vi "Puzzle 3-2.vi"() -> ()   [LabVIEW 2022 SP3]
panel:
  out "Array 4":cluster{i32, i32}[](array[cluster])
  out "sum":i32
  out "Array 3":cluster{i32, i32}[](array[cluster])
  out "Array 2":enum16{"Letter", "Number", "Symbol", "Dot"}[][](array[ring])
  out "Array":string[][](array[string])
  in  "delimited string":string
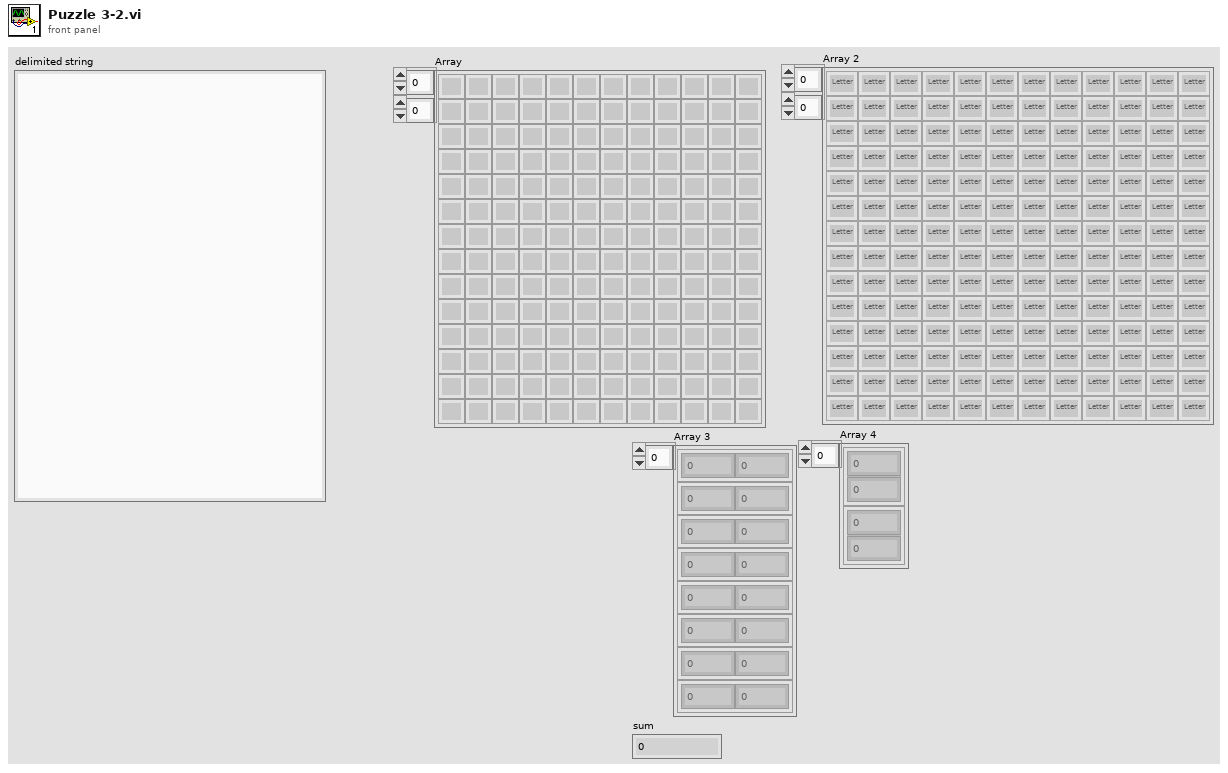
[diagram p1: front panel]
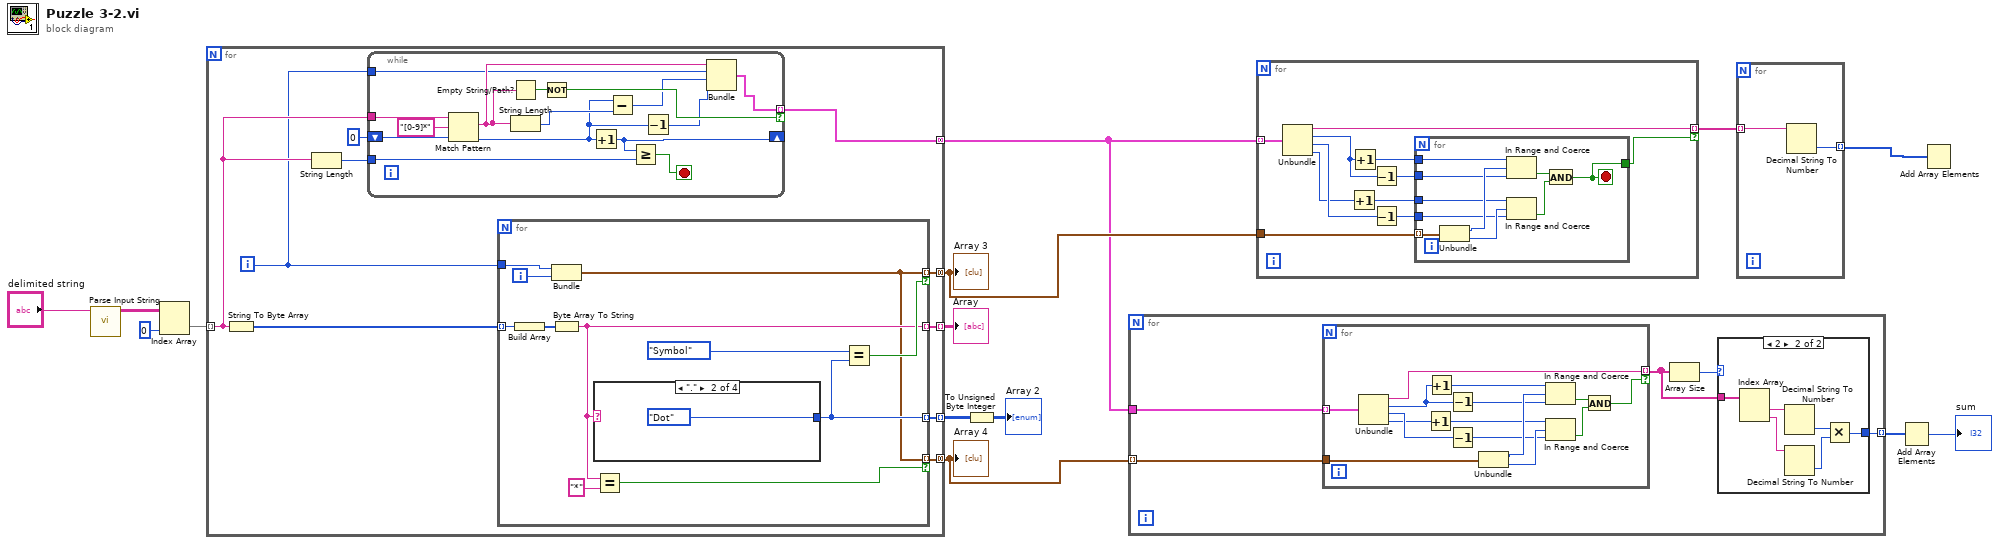
[diagram p0: block diagram]
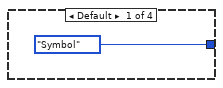
[diagram p3: hidden frame]
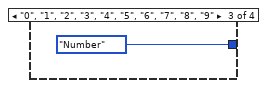
[diagram p4: hidden frame]
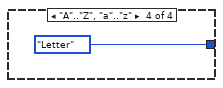
[diagram p5: hidden frame]
diagram:
  n1 = call "Parse Input String.vi"("delimited string"="delimited string") -> ("parsed string"=w13:string[][])  [unwired: 10 in]
  n2 = Index Array(array=w13, index (col)=0 ("disabled index (col)")) -> (element=w11:string[])  [unwired: 1 in]
  n3 = for {
    tunnel: w11 -> [w19] mode=indexing
    tunnel: [w23] -> w10 mode=indexing
    tunnel: [w22] -> w9 mode=indexing
    tunnel: [w21] -> w7 mode=concatenating
    tunnel: [w16] -> w3 mode=concatenating
    tunnel: [w15] -> w4 mode=concatenating
    i -> [w17]
    n4 = String To Byte Array(string=w19) -> (unsigned byte array=w24:u8[])
    n5 = String Length(string=w19) -> (length=w18:i32)
    n6 = while {
      tunnel: w19 -> [w38]
      tunnel: [w26] -> w16 mode=indexing if=w39
      shift-right: [w32] -> _
      shift-left: 0 -> [w37]
      tunnel: w18 -> [w35]
      tunnel: w17 -> [w25]
      stop <- w33 stop-if-true
      n7 = Match Pattern(string=w38, regular expression="[0-9]*" ("format string"), offset (0)=w37) -> (match substring=w30:string, offset past match=w28:i32)  [unwired: 2 out]
      n8 = Empty String/Path?(string/path=w30) -> (empty?=w34:bool)
      n9 = String Length(string=w30) -> (length=w31:i32)
      n10 = Not(x=w34) -> (.not. x?=w39:bool)
      n11 = Increment(x=w28) -> (x+1=w32:i32)
      n12 = Subtract(x=w28, y=w31) -> (x-y=w29:i32)
      n13 = Greater Or Equal?(x=w32, y=w35) -> (x >= y?=w33:bool)
      n14 = Decrement(x=w28) -> (x-1=w27:i32)
      n15 = Bundle(w30, w25, w29, w27) -> (w26:cluster{string, i32, i32, i32})  [unwired: 1 in]
    }
    n16 = for {
      tunnel: w24 -> [w50] mode=indexing
      tunnel: [w43] -> w23 mode=indexing
      tunnel: [w48] -> w22 mode=indexing
      tunnel: w17 -> [w45]
      tunnel: [w41] -> w21 mode=indexing if=w44
      tunnel: [w41] -> w15 mode=indexing if=w40
      i -> [w46]
      n17 = Build Array(w50) -> (w49:u8[])
      n18 = Bundle(w45, w46) -> (w41:cluster{i32, i32})  [unwired: 1 in]
      n19 = Byte Array To String(unsigned byte array=w49) -> (string=w43:string)
      n20 = case shown="\".\"" w43 {
        tunnel: [enum16{"Letter", "Number", "Symbol", "Dot"}."Symbol" enum16{"Letter", "Number", "Symbol", "Dot"}."Dot" enum16{"Letter", "Number", "Symbol", "Dot"}."Number" enum16{"Letter", "Number", "Symbol", "Dot"}."Letter"] -> w48
        frame Default {
        }
        frame "." {
        }
        frame "0", "1", "2", "3", "4", "5", "6", "7", "8", "9" {
        }
        frame "A".."Z", "a".."z" {
        }
      }
      n21 = Equal?(x=w43, y="*") -> (x = y?=w40:bool)
      n22 = Equal?(x=enum16{"Letter", "Number", "Symbol", "Dot"}."Symbol", y=w48) -> (x = y?=w44:bool)
    }
  }
  "Array" <- w10
  "Array 3" <- w7
  "Array 4" <- w4
  n23 = To Unsigned Byte Integer(number=w9) -> (unsigned 8bit integer=→"Array 2":u8[][])
  n24 = for {
    tunnel: w4 -> [w58] mode=indexing
    tunnel: w3 -> [w59]
    tunnel: [w55] -> w2 mode=indexing
    n25 = for {
      tunnel: w58 -> [w80]
      tunnel: w59 -> [w68] mode=indexing
      tunnel: [w67] -> w56 mode=indexing if=w66
      n26 = Unbundle(w68) -> (w67:string, w75:i32, w74:i32, w73:i32)
      n27 = Increment(x=w73) -> (x+1=w72:i32)
      n28 = Increment(x=w75) -> (x+1=w71:i32)
      n29 = Decrement(x=w75) -> (x-1=w70:i32)
      n30 = Decrement(x=w74) -> (x-1=w69:i32)
      n31 = Unbundle(w80) -> (w79:i32, w78:i32)
      n32 = In Range and Coerce(upper limit=w71, x=w79, lower limit=w70) -> (In Range?=w77:bool)  [unwired: 1 out]
      n33 = In Range and Coerce(upper limit=w72, x=w78, lower limit=w69) -> (In Range?=w76:bool)  [unwired: 1 out]
      n34 = And(x=w77, y=w76) -> (x .and. y?=w66:bool)
    }
    n35 = Array Size(array=w56) -> (size(s)=w57:i32)
    n36 = case shown="2" w57 {
      tunnel: w56 -> [_ w65]
      tunnel: [_ w60] -> w55
      frame Default {
      }
      frame 2 {
        n37 = Index Array(array=w65) -> (element #1=w64:string, element #2=w63:string)  [unwired: 2 in]
        n38 = Decimal String To Number(string=w64) -> (number=w62:i32)  [unwired: 2 in, 1 out]
        n39 = Decimal String To Number(string=w63) -> (number=w61:i32)  [unwired: 2 in, 1 out]
        n40 = Multiply(x=w62, y=w61) -> (x*y=w60:i32)
      }
    }
  }
  n41 = for {
    tunnel: w3 -> [w91] mode=indexing
    tunnel: w7 -> [w87]
    tunnel: [w81] -> w6 mode=indexing if=w82
    n42 = Unbundle(w91) -> (w81:string, w90:i32, w89:i32, w88:i32)
    n43 = Increment(x=w88) -> (x+1=w84:i32)
    n44 = Increment(x=w90) -> (x+1=w85:i32)
    n45 = Decrement(x=w90) -> (x-1=w86:i32)
    n46 = Decrement(x=w89) -> (x-1=w83:i32)
    n47 = for {
      tunnel: w87 -> [w101] mode=indexing
      tunnel: w86 -> [w98]
      tunnel: w85 -> [w97]
      tunnel: w84 -> [w96]
      tunnel: w83 -> [w95]
      tunnel: [w92] -> w82
      stop <- w92 stop-if-true
      n48 = Unbundle(w101) -> (w100:i32, w99:i32)
      n49 = In Range and Coerce(upper limit=w97, x=w100, lower limit=w98) -> (In Range?=w94:bool)  [unwired: 1 out]
      n50 = In Range and Coerce(upper limit=w96, x=w99, lower limit=w95) -> (In Range?=w93:bool)  [unwired: 1 out]
      n51 = And(x=w94, y=w93) -> (x .and. y?=w92:bool)
    }
  }
  n52 = for {
    tunnel: w6 -> [w103] mode=indexing
    tunnel: [w102] -> w5 mode=indexing
    n53 = Decimal String To Number(string=w103) -> (number=w102:i32)  [unwired: 2 in, 1 out]
  }
  n54 = Add Array Elements(numeric array=w2) -> (sum=→"sum":i32)
  n55 = Add Array Elements(numeric array=w5) -> ()  [unwired: 1 out]
